vi "Add Nonzero Time Property.vi"(7 "Property":string, 10 "Time Stamp":timestamp, 11 "String in":string) -> (3 "String":string)   [LabVIEW 2020, in "JWT.lvlib" / "JWT.lvclass"]
uses:
  JWT.lvclass
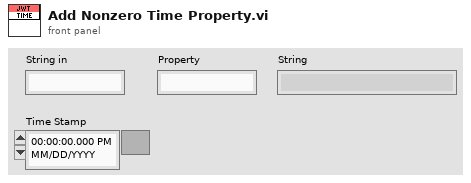
[diagram p1: front panel]
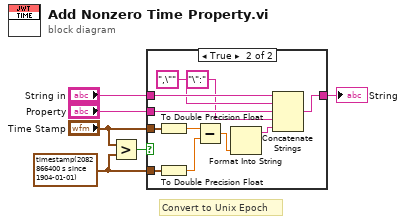
[diagram p0: block diagram]
diagram:
  w1 = timestamp(2082866400 s since 1904-01-01) ("Time Stamp")
  # "Convert to Unix Epoch"
  n1 = Greater?(x="Time Stamp", y=w1) -> (0:w6:bool)
  n2 = case shown="True" w6 {
    tunnel: "Time Stamp" -> [_ w18]
    tunnel: "String in" -> [w7 w16]
    tunnel: [w7 w15] -> w3
    tunnel: "Property" -> [_ w13]
    tunnel: w1 -> [_ w10]
    frame False {
    }
    frame True {
      n3 = To Double Precision Float(number=w18) -> (double precision float=w17:dbl)
      n4 = To Double Precision Float(number=w10) -> (double precision float=w8:dbl)
      n5 = Subtract(x=w17, y=w8) -> (x-y=w9:dbl)
      n6 = Format Into String(w9) -> (resulting string=w11:string)  [unwired: 3 in, 1 out]
      n7 = Concatenate Strings(w16, ",\"" ("string"), w13, "\":" ("string"), w11) -> (w15:string)
    }
  }
  "String" <- w3
